vi "read_all_waveforms.vi"(8 "error in (no error)":errorcluster, 10 "Small?":bool, 11 "Dust Event ID":i32) -> (0 "error out":errorcluster, 1 "Offset Array":dbl[](array[numeric]), 2 "dt":dbl, 3 "Waveform":T1)   [LabVIEW 2013]
uses:
  Database2.0/Private/Controls/Waveforms.ctl
  <vilib>/addons/h5labview/H5F_mode.ctl
  Database2.0/Public API/Post_Signal.ctl
  Database2.0/Private/Controls/Role ID.ctl
  Database2.0/Private/Controls/Hardware ID.ctl
  <userlib>/_OpenG.lib/file/file.llb/File Exists - Scalar__ogtk.vi
  <vilib>/addons/h5labview/polymorph/H5A_read_var.vi
  <vilib>/addons/database/_DB Variant To Data/Database Variant To Data.xnode
  <vilib>/addons/h5labview/H5File.lvlib
  <vilib>/addons/h5labview/H5GroupObject.lvlib
  <vilib>/addons/h5labview/H5Attrib.lvlib
panel:
  out "Query Syntax":string
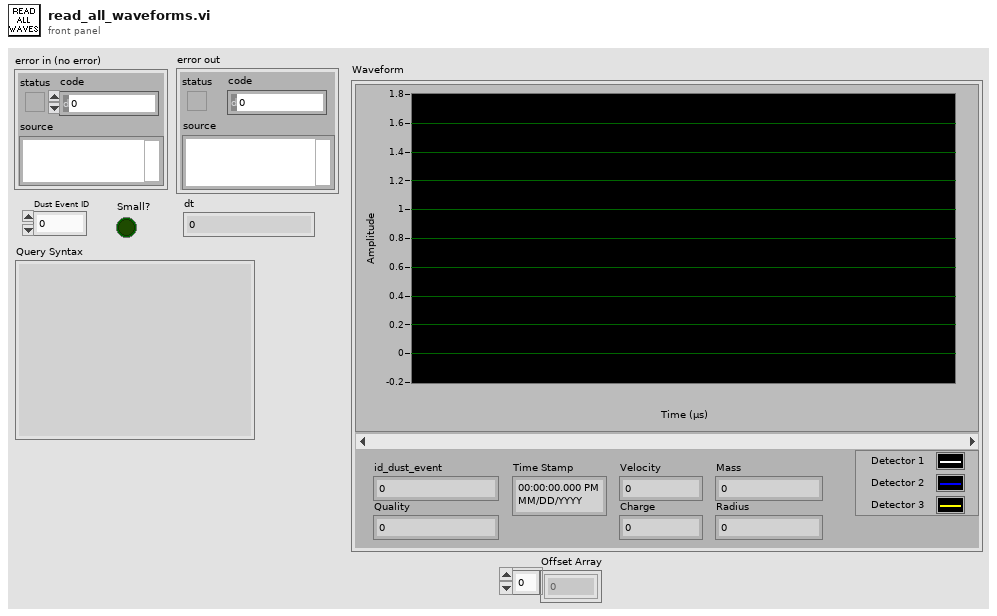
[diagram p1: front panel]
types:
  T1 = typedef "Waveforms.ctl" = cluster{"id_dust_event":u64, "Time Stamp":timestamp, "Velocity":dbl, "Mass":dbl, "Charge":dbl, "Radius":dbl, "Waveform Graph":sgl[][], "Quality":i32}
  T2 = typedef "H5File.lvlib/H5F_mode.ctl" = enum16{"read-only", "read-write", "overwrite", "create new", "open or create"}
  T3 = typedef "Role ID.ctl" = enum16{"First_Detector", "Second_Detector", "Third_Detector", "LeCroy_CH1", "LeCroy_CH2", "LeCroy_CH3", "LeCroy_CH4", "PSU"}
  T4 = typedef "Post_Signal.ctl" = cluster{"Integer Timestamp":i64, "Dust Event ID":i64, "Role ID":T3, "Data":sgl[], "Signal Length":i32, "dt":sgl, "Offset":dbl, "Hardware ID":T5}
  T5 = typedef "Hardware ID.ctl" = enum16{"Unknown", "CSA 1", "CSA 2", "CSA 3", "CSA 4", "CSA 5", "CSA 6"}
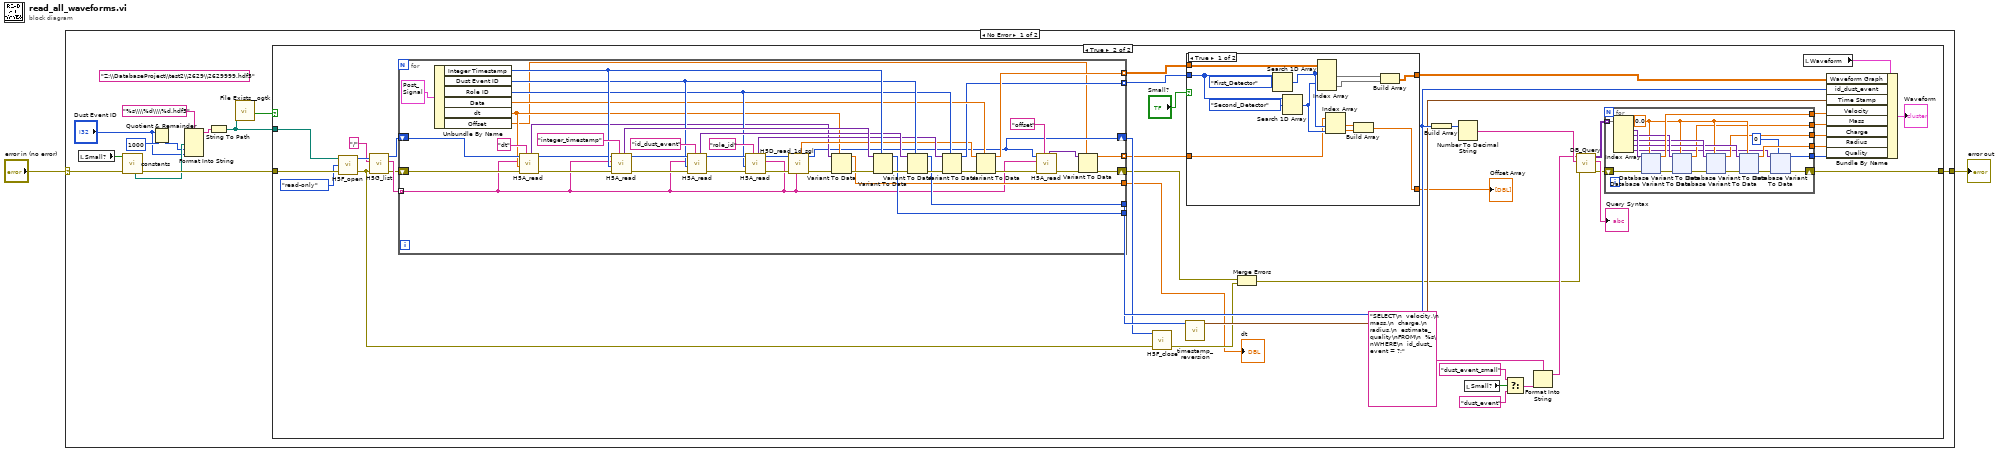
[diagram p0: block diagram]
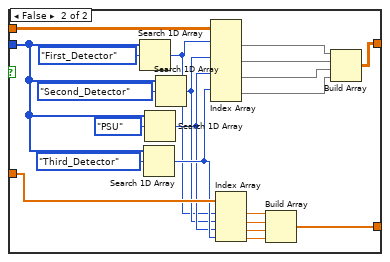
[diagram p3: hidden frame]
diagram:
  n1 = case shown="No Error" "error in (no error)" {
    selector: "error in (no error)" -> [w13 w315]
    tunnel: [w6 w315] -> w1
    frame No Error {
      (unwired) "Z:\\DatabaseProject\\test2\\2629\\2629999.hdf5"
      n2 = local read "Small?"() -> (w7:bool)
      n3 = call "constants.vi"("error in (no error)"=w13, "Small?"=w7) -> ("error out"=w14:errorcluster, "file path for Processed Signal .hdf5 files"=w10:path)  [unwired: 4 in, 4 out]
      n4 = Quotient & Remainder(x="Dust Event ID", y=1000) -> (floor(x/y)=w9:i32)  [unwired: 1 out]
      n5 = Format Into String(format string="%s\\\\%d\\\\%d.hdf5", w10, w9, "Dust Event ID") -> (resulting string=w3:string)  [unwired: 2 in, 1 out]
      n6 = String To Path(string=w3) -> (path=w4:path)
      n7 = call-poly <userlib>:"File Exists__ogtk.vi"("file path"=w4) -> ("exists"=w5:bool)  [unwired: 6 in, 1 out]
      n8 = case shown="True" w5 {
        tunnel: w14 -> [w15 w57]
        tunnel: w4 -> [_ w56]
        tunnel: [w15 w54] -> w6
        frame False {
        }
        frame True {
          n9 = call <vilib>:"H5F_open.vi"("error in (no error)"=w57, "mode"=H5F_mode."read-only", "path"=w56) -> ("error out"=w21:errorcluster, "ref"=w53:i32)  [unwired: 1 in]
          n10 = call <vilib>:"H5G_list.vi"("error in (no error)"=w21, "group"="/", "ref"=w53) -> ("error out"=w25:errorcluster, "names"=w29:string[], "ref out"=w26:i32)  [unwired: 1 in, 1 out]
          n11 = for {
            shift-right: [w273] -> w19
            shift-left: w25 -> [w287]
            shift-right: [w276] -> w27
            shift-left: w26 -> [w289]
            tunnel: w29 -> [w278] mode=indexing
            tunnel: [w293] -> w31 mode=indexing
            tunnel: [w294] -> w32 mode=indexing
            tunnel: [w291] -> w50
            tunnel: [w292] -> w33
            tunnel: [w282] -> w18
            tunnel: [w271] -> w17 mode=indexing
            n12 = Unbundle By Name(T4 {"Integer Timestamp"=0, "Dust Event ID"=0, "Role ID"=enum."First_Detector", "Data"=[], "Signal Length"=0, "dt"=0.0, "Offset"=0.0, "Hardware ID"=enum."CSA 1"} ("Post_Signal 2")) -> ("Integer Timestamp"=w312:i64, "Dust Event ID"=w306:i64, "Role ID"=w300:T3, "Data"=w297:sgl[], "dt"=w280:sgl, "Offset"=w272:dbl)
            n13 = call-poly <vilib>:"H5A_read.vi"("attrib_name"="dt", "error in (no error)"=w287, "default"=w280, "obj_name"=w278, "ref"=w289) -> ("error out"=w286:errorcluster, "ref out"=w288:i32, "value"=w283:variant)  [unwired: 2 in]
            n14 = call-poly <vilib>:"H5A_read.vi"("attrib_name"="integer_timestamp", "error in (no error)"=w286, "default"=w312, "obj_name"=w278, "ref"=w288) -> ("error out"=w308:errorcluster, "ref out"=w310:i32, "value"=w311:variant)  [unwired: 2 in]
            n15 = call-poly <vilib>:"H5A_read.vi"("attrib_name"="id_dust_event", "error in (no error)"=w308, "default"=w306, "obj_name"=w278, "ref"=w310) -> ("error out"=w304:errorcluster, "ref out"=w303:i32, "value"=w307:variant)  [unwired: 2 in]
            n16 = call-poly <vilib>:"H5A_read.vi"("attrib_name"="role_id", "error in (no error)"=w304, "default"=w300, "obj_name"=w278, "ref"=w303) -> ("error out"=w295:errorcluster, "ref out"=w296:i32, "value"=w301:variant)  [unwired: 2 in]
            n17 = call "H5D_read_1d_sgl.vi"("name"=w278, "error in (no error)"=w295, "ref"=w296) -> ("error out"=w285:errorcluster, "ref out"=w276:i32, "data"=w290:sgl[])  [unwired: 4 in]
            n18 = Variant To Data(error in=w285, type=w280, Variant=w283) -> (data=w282:sgl, error out=w284:errorcluster)
            n19 = Variant To Data(error in=w284, type=w312, Variant=w311) -> (data=w292:i64, error out=w305:errorcluster)
            n20 = Variant To Data(error in=w305, type=w306, Variant=w307) -> (data=w291:i64, error out=w299:errorcluster)
            n21 = Variant To Data(error in=w299, type=w300, Variant=w301) -> (data=w293:T3, error out=w298:errorcluster)
            n22 = Variant To Data(error in=w298, type=w297, Variant=w290) -> (data=w294:sgl[], error out=w279:errorcluster)
            n23 = call-poly <vilib>:"H5A_read.vi"("attrib_name"="offset", "error in (no error)"=w279, "obj_name"=w278, "ref"=w276) -> ("error out"=w274:errorcluster, "value"=w275:variant)  [unwired: 3 in, 1 out]
            n24 = Variant To Data(error in=w274, type=w272, Variant=w275) -> (data=w271:dbl, error out=w273:errorcluster)
          }
          "dt" <- w18
          n25 = call <vilib>:"H5F_close.vi"("error in (no error)"=w21, "ref"=w27) -> ("error out"=w22:errorcluster)  [unwired: 3 in]
          n26 = call "timestamp_reversion.vi"("Integer Timestamp"=w33) -> ("time stamp"=w34:timestamp)  [unwired: 8 in, 1 out]
          n27 = case shown="True" "Small?" {
            tunnel: w31 -> [w247 w263]
            tunnel: w32 -> [w246 w267]
            tunnel: [w244 w266] -> w23
            tunnel: w17 -> [w240 w259]
            tunnel: [w237 w250] -> w16
            frame True {
              n28 = Search 1D Array(1D array=w247, element=Role_ID."First_Detector") -> (index of element=w242:i32)  [unwired: 1 in]
              n29 = Search 1D Array(1D array=w247, element=Role_ID."Second_Detector") -> (index of element=w241:i32)  [unwired: 1 in]
              n30 = Index Array(array=w246, index (row) #1=w242, index (row) #2=w241) -> (element #1=w243:sgl[], element #2=w245:sgl[])  [unwired: 2 in]
              n31 = Index Array(array=w240, index #1=w242, index #2=w241) -> (element #1=w239:dbl, element #2=w238:dbl)
              n32 = Build Array(w239, w238) -> (w237:dbl[])
              n33 = Build Array(w243, w245) -> (w244:sgl[][])
            }
            frame False {
              n34 = Search 1D Array(1D array=w263, element=Role_ID."First_Detector") -> (index of element=w255:i32)  [unwired: 1 in]
              n35 = Search 1D Array(1D array=w263, element=Role_ID."Third_Detector") -> (index of element=w258:i32)  [unwired: 1 in]
              n36 = Search 1D Array(1D array=w263, element=Role_ID."PSU") -> (index of element=w257:i32)  [unwired: 1 in]
              n37 = Search 1D Array(1D array=w263, element=Role_ID."Second_Detector") -> (index of element=w256:i32)  [unwired: 1 in]
              n38 = Index Array(array=w267, index (row) #1=w255, index (row) #2=w256, index (row) #3=w257, index (row) #4=w258) -> (element #1=w261:sgl[], element #2=w260:sgl[], element #3=w265:sgl[], element #4=w262:sgl[])  [unwired: 4 in]
              n39 = Index Array(array=w259, index #1=w255, index #2=w256, index #3=w257, index #4=w258) -> (element #1=w254:dbl, element #2=w253:dbl, element #3=w252:dbl, element #4=w251:dbl)
              n40 = Build Array(w254, w253, w252, w251) -> (w250:dbl[])
              n41 = Build Array(w261, w260, w265, w262) -> (w266:sgl[][])
            }
          }
          "Offset Array" <- w16
          n42 = Merge Errors(w19, w22) -> (w20:errorcluster)
          n43 = Build Array(w50) -> (w51:i64[])
          n44 = Number To Decimal String(number=w51) -> (decimal integer string=w52:string[])  [unwired: 1 in]
          n45 = local read "Small?"() -> (w38:bool)
          n46 = Select(t="dust_event_small" ("resulting string"), s=w38, f="dust_event" ("resulting string")) -> (s? t:f=w37:string)
          n47 = Format Into String(format string="SELECT\n  velocity,\n  mass,\n  charge,\n  radius,\n  estimate_quality\nFROM\n  %s\nWHERE\n  id_dust_event = ?;" ("SQL query"), w37) -> (resulting string=w49:string)  [unwired: 2 in, 1 out]
          n48 = call "DB_Query.vi"("error in (no error)"=w20, "Parameters"=w52, "Parameterized Query"=w49) -> ("error out"=w46:errorcluster, "Query in Standard Format"=→"Query Syntax":string, "Results"=w47:variant[][])  [unwired: 6 in]
          n49 = for {
            tunnel: w47 -> [w75] mode=indexing
            shift-right: [w61] -> w54
            shift-left: w46 -> [w76]
            tunnel: [w72] -> w41
            tunnel: [w65] -> w42
            tunnel: [w64] -> w43
            tunnel: [w63] -> w44
            tunnel: [w58] -> w45
            w66 = 0.0 ("Velocity")
            n50 = Index Array(array=w75) -> (element #1=w74:variant, element #2=w71:variant, element #3=w69:variant, element #4=w67:variant, element #5=w60:variant)  [unwired: 5 in]
            n51 = xnode "Database Variant To Data"("database variant"=w74, "error in (no error)"=w76, "type"=w66) -> ("data"=w72:dbl, "error out"=w73:errorcluster)
            n52 = xnode "Database Variant To Data"("database variant"=w71, "error in (no error)"=w73, "type"=w66) -> ("data"=w65:dbl, "error out"=w70:errorcluster)
            n53 = xnode "Database Variant To Data"("database variant"=w69, "error in (no error)"=w70, "type"=w66) -> ("data"=w64:dbl, "error out"=w68:errorcluster)
            n54 = xnode "Database Variant To Data"("database variant"=w67, "error in (no error)"=w68, "type"=w66) -> ("data"=w63:dbl, "error out"=w62:errorcluster)
            n55 = xnode "Database Variant To Data"("database variant"=w60, "error in (no error)"=w62, "type"=i64 0 ("Dust Event ID")) -> ("data"=w58:i64, "error out"=w61:errorcluster)
          }
          n56 = local read "Waveform"() -> (w30:T1)
          n57 = Bundle By Name(cluster=w30, "Waveform Graph"=w23, "id_dust_event"=w50, "Time Stamp"=w34, "Velocity"=w41, "Mass"=w42, "Charge"=w43, "Radius"=w44, "Quality"=w45) -> (→"Waveform":T1)
        }
      }
    }
    frame Error {
    }
  }
  "error out" <- w1
